vi "Calculate MC delay.vi"(10 "Cycles to wait after trigger":u16, 11 "AOD Fill":u16) -> (3 "mc delay prog read":u16)   [LabVIEW 2020]
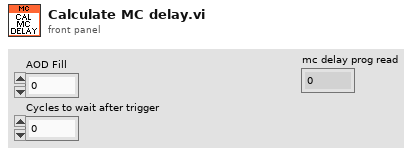
[diagram p1: front panel]
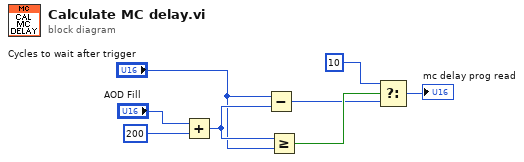
[diagram p0: block diagram]
diagram:
  n1 = Add(x="AOD Fill", y=u16 200) -> (x+y=w6:u16)
  n2 = Subtract(x="Cycles to wait after trigger", y=w6) -> (x-y=w2:u16)
  n3 = Greater Or Equal?(x=w6, y="Cycles to wait after trigger") -> (x >= y?=w4:bool)
  n4 = Select(t=u16 10, s=w4, f=w2) -> (s? t:f=→"mc delay prog read":u16)
